vi "SaveData.vi"(0 "object in":refnum<class "Application.lvclass">, 5 "error in (no error)":errorcluster) -> (14 "object out":refnum<class "Application.lvclass">, 19 "error out":errorcluster)   [LabVIEW 2023, in "Application.lvclass"]
uses:
  Application.lvclass
  TDMSLogger_PowerScan_class/TDMSLogger_PowerScan.lvclass
  MTEC_Async_class/MTEC_Async.lvclass
  InstrumentBase_class/AD2_SDK_class/InstrumentBase.lvclass
  CetoniPump_class/CetoniPump.lvclass
  Hamamatsu_class/Hamamatsu.lvclass
  Application.lvclass/Application.ctl
panel:
  in  "group name in (Untitled)":string
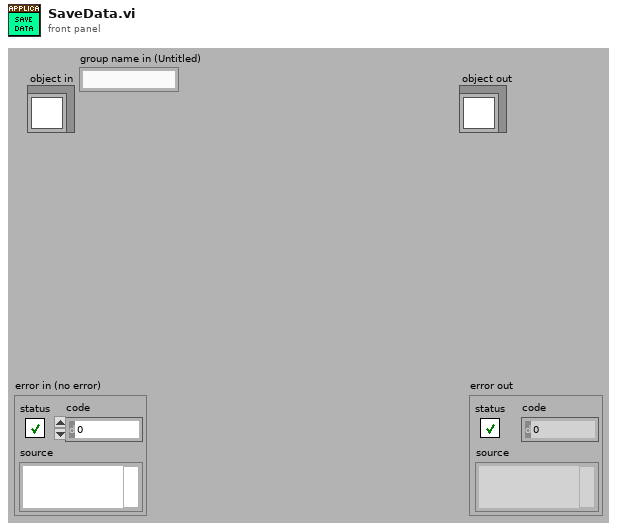
[diagram p1: front panel]
types:
  T1 = typedef "meTEC_ID 1200_Temperature is Stable.ctl" = i32
  T2 = typedef "meTEC_ID 104_Device Status.ctl" = i32
  T3 = cluster{"current time":timestamp, "DataOut":cluster{"meTEC_CH2_Temperature Stability":T1, "meTEC_CH2_Act. Output Current [A]":dbl, "meTEC_CH2_Act. Output Voltage [V]":dbl, "meTEC_CH2_Object Temperature [°C]":dbl, "meTEC_CH2_Sink Temperature [°C]":dbl, "meTEC_CH1_Error Parameter":i32, "meTEC_CH1_Error Instance":i32, "meTEC_CH1_Error No.":i32, "meTEC_CH1_Device Status":T2, "meTEC_CH1_Temperature Stability":T1, "meTEC_CH1_Act. Output Current [A]":dbl, "meTEC_CH1_Act. Output Voltage [V]":dbl, "meTEC_CH1_Object Temperature [°C]":dbl, "meTEC_CH1_Sink Temperature [°C]":dbl}}[]
  T4 = typedef "IMAQ Image.ctl" = refnum<image>
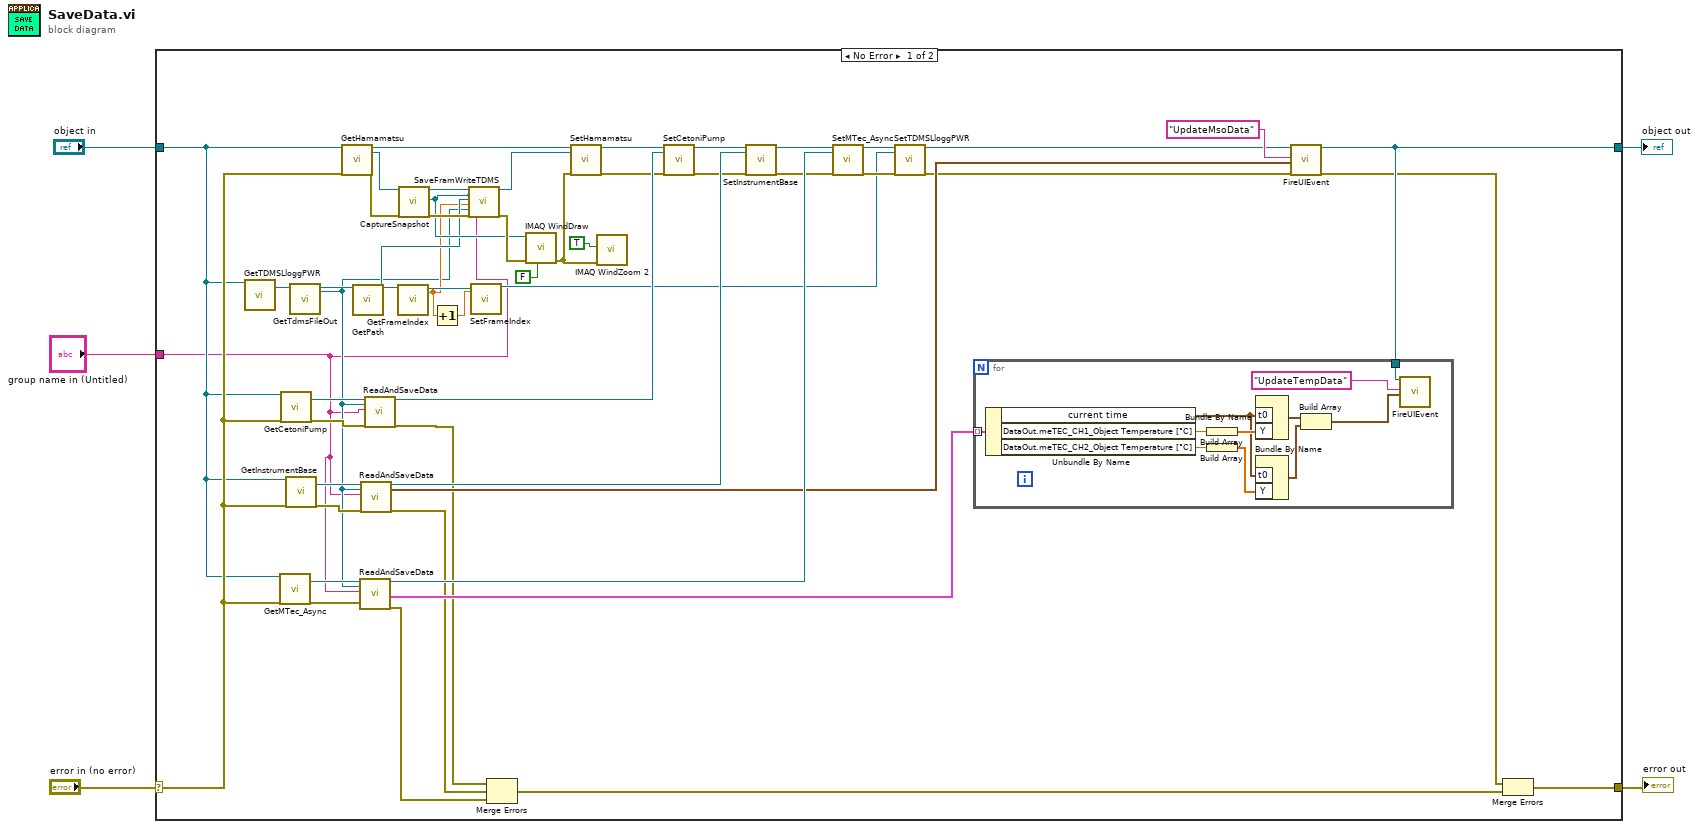
[diagram p0: block diagram]
diagram:
  n1 = case shown="No Error" "error in (no error)" {
    selector: "error in (no error)" -> [w32 w70]
    tunnel: [w26 w70] -> w4
    tunnel: [w51 w69] -> w2
    tunnel: "object in" -> [w24 w69]
    tunnel: "group name in (Untitled)" -> [w6 _]
    frame No Error {
      n2 = call-dynamic "GetTDMSLloggPWR.vi"("object in"=w24) -> ("TDMSLloggPWR"=w23:refnum<class "TDMSLogger_PowerScan.lvclass">)  [unwired: 16 in, 2 out]
      n3 = call-dynamic "GetMTec_Async.vi"("object in"=w24, "error in (no error)"=w32) -> ("MTec_Async"=w41:refnum<class "MTEC_Async.lvclass">, "error out"=w38:errorcluster)  [unwired: 15 in, 1 out]
      n4 = call-dynamic "GetCetoniPump.vi"("object in"=w24, "error in (no error)"=w32) -> ("CetoniPump"=w49:refnum<class "CetoniPump.lvclass">, "error out"=w40:errorcluster)  [unwired: 15 in, 1 out]
      n5 = call-dynamic "GetInstrumentBase.vi"("object in"=w24, "error in (no error)"=w32) -> ("InstrumentBase"=w50:refnum<class "InstrumentBase.lvclass">, "error out"=w39:errorcluster)  [unwired: 15 in, 1 out]
      n6 = call-dynamic "GetTdmsFileOut.vi"("object in"=w23) -> ("object out"=w14:refnum<class "TDMSLogger_PowerScan.lvclass">, "tdms file out"=w7:refnum<k34>)  [unwired: 16 in, 1 out]
      n7 = call-dynamic "GetHamamatsu.vi"("object in"=w24, "error in (no error)"=w32) -> ("object out"=w57:refnum<class "Application.lvclass">, "Hamamatsu"=w56:refnum<class "Hamamatsu.lvclass">, "error out"=w55:errorcluster)  [unwired: 15 in]
      n8 = call-dynamic "GetPath.vi"("object in"=w14) -> ("object out"=w12:refnum<class "TDMSLogger_PowerScan.lvclass">, "Path"=w13:path)  [unwired: 16 in, 1 out]
      n9 = call-dynamic "ReadAndSaveData.vi"("object in"=w41, "tdms file"=w7, "group name in (Untitled)"=w6, "error in (no error)"=w38) -> ("object out"=w37:refnum<class "MTEC_Async.lvclass">, "Buffer"=w34:T3, "error out"=w28:errorcluster)  [unwired: 12 in, 1 out]
      n10 = call-dynamic "ReadAndSaveData.vi"("object in"=w50, "tdms file"=w7, "group name in (Untitled)"=w6, "error in (no error)"=w39) -> ("object out"=w45:refnum<class "InstrumentBase.lvclass">, "Channels array"=w33:waveform(dbl)[], "error out"=w29:errorcluster)  [unwired: 12 in, 1 out]
      n11 = call-dynamic "ReadAndSaveData.vi"("object in"=w49, "tdms file"=w7, "group name in (Untitled)"=w6, "error in (no error)"=w40) -> ("object out"=w48:refnum<class "CetoniPump.lvclass">, "error out"=w30:errorcluster)  [unwired: 14 in]
      n12 = call-dynamic "GetFrameIndex.vi"("object in"=w12) -> ("object out"=w11:refnum<class "TDMSLogger_PowerScan.lvclass">, "FrameIndex"=w10:dbl)  [unwired: 16 in, 1 out]
      n13 = call-dynamic "CaptureSnapshot.vi"("object in"=w56, "error in (no error)"=w55) -> ("object out"=w22:refnum<class "Hamamatsu.lvclass">, "FreeRunningImage"=w18:T4, "error out"=w20:errorcluster)  [unwired: 14 in, 1 out]
      n14 = Increment(x=w10) -> (x+1=w9:dbl)
      n15 = call-dynamic "SaveFramWriteTDMS.vi"("object in"=w22, "Image"=w18, "base path"=w13, "FrameIdx"=w10, "tdms file"=w7, "error in (no error)"=w20, "group name"=w6) -> ("object out"=w21:refnum<class "Hamamatsu.lvclass">, "error out"=w19:errorcluster)  [unwired: 11 in]
      n16 = call-dynamic "SetFrameIndex.vi"("object in"=w11, "FrameIndex"=w9) -> ("object out"=w8:refnum<class "TDMSLogger_PowerScan.lvclass">)  [unwired: 16 in, 1 out]
      n17 = Merge Errors(w30, w29, w28) -> (w27:errorcluster)
      n18 = call "IMAQ WindDraw"("Resize to Image Size? (Y)"=FALSE, "error in (no error)"=w19, "Image"=w18) -> ("error out"=w25:errorcluster)  [unwired: 7 in, 1 out]
      n19 = call-dynamic "SetHamamatsu.vi"("object in"=w57, "Hamamatsu"=w21, "error in (no error)"=w25) -> ("object out"=w47:refnum<class "Application.lvclass">, "error out"=w44:errorcluster)  [unwired: 15 in]
      n20 = call "IMAQ WindZoom 2"("error in (no error)"=w25, "Zoom to Fit? (False)"=TRUE) -> ()  [unwired: 6 in, 4 out]
      n21 = call-dynamic "SetCetoniPump.vi"("object in"=w47, "CetoniPump"=w48, "error in (no error)"=w44) -> ("object out"=w46:refnum<class "Application.lvclass">, "error out"=w43:errorcluster)  [unwired: 15 in]
      n22 = call-dynamic "SetInstrumentBase.vi"("object in"=w46, "InstrumentBase"=w45, "error in (no error)"=w43) -> ("object out"=w42:refnum<class "Application.lvclass">, "error out"=w36:errorcluster)  [unwired: 15 in]
      n23 = call-dynamic "SetMTec_Async.vi"("object in"=w42, "MTec_Async"=w37, "error in (no error)"=w36) -> ("object out"=w35:refnum<class "Application.lvclass">, "error out"=w16:errorcluster)  [unwired: 15 in]
      n24 = call-dynamic "SetTDMSLloggPWR.vi"("object in"=w35, "TDMSLloggPWR"=w8, "error in (no error)"=w16) -> ("object out"=w17:refnum<class "Application.lvclass">, "error out"=w15:errorcluster)  [unwired: 15 in]
      n25 = call-dynamic "FireUIEvent.vi"("object in"=w17, "Message"="UpdateMsoData", "Message Data"=w33, "error in (no error)"=w15) -> ("object out"=w51:refnum<class "Application.lvclass">, "error out"=w31:errorcluster)  [unwired: 14 in]
      n26 = for {
        tunnel: w34 -> [w60] mode=indexing
        tunnel: w51 -> [w58]
        n27 = Unbundle By Name(w60) -> ("current time"=w65:timestamp, "DataOut.meTEC_CH1_Object Temperature [°C]"=w64:dbl, "DataOut.meTEC_CH2_Object Temperature [°C]"=w62:dbl)
        n28 = Build Array(w64) -> (w66:dbl[])
        n29 = Build Array(w62) -> (w63:dbl[])
        n30 = Bundle By Name("t0"=w65, "Y"=w66) -> (w68:waveform(dbl))  [unwired: 1 in]
        n31 = Bundle By Name("t0"=w65, "Y"=w63) -> (w67:waveform(dbl))  [unwired: 1 in]
        n32 = Build Array(w68, w67) -> (w59:waveform(dbl)[])
        n33 = call-dynamic "FireUIEvent.vi"("object in"=w58, "Message"="UpdateTempData", "Message Data"=w59) -> ()  [unwired: 15 in, 2 out]
      }
      n34 = Merge Errors(w31, w27) -> (w26:errorcluster)
    }
    frame Error {
    }
  }
  "error out" <- w4
  "object out" <- w2
